vi "FP_Size To Bounds.vi"(8 "Error":errorcluster, 9 "Border Spacing":i16, 10 "Bounds":T2, 11 "VI":refnum<vi>) -> (0 "Error Out":errorcluster, 2 "Front Panel box":T1, 3 "VI Out":refnum<vi>)   [LabVIEW 2024]
uses:
  <vilib>/Utility/miscctls.llb/LVBoundsTypeDef.ctl
  <vilib>/Utility/miscctls.llb/LVRectTypeDef.ctl
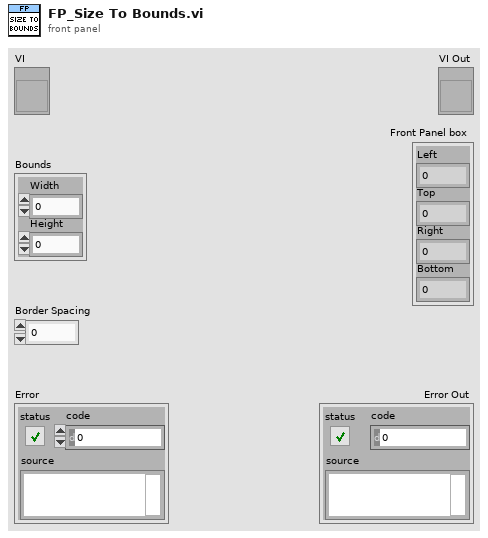
[diagram p1: front panel]
types:
  T1 = typedef "LVRectTypeDef.ctl" = cluster{"Left":i16, "Top":i16, "Right":i16, "Bottom":i16}
  T2 = typedef "LVBoundsTypeDef.ctl" = cluster{"Width":u32, "Height":u32}
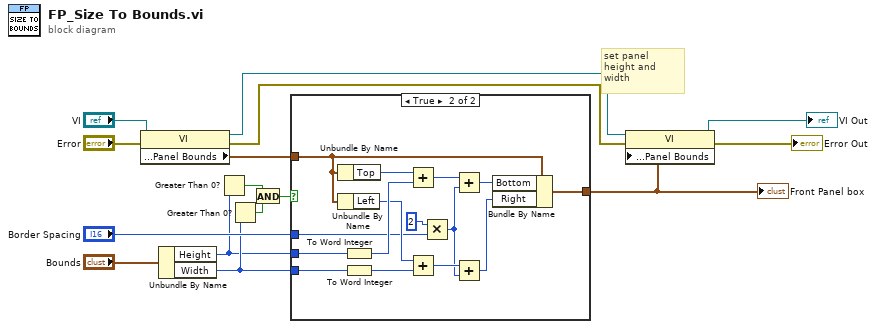
[diagram p0: block diagram]
diagram:
  # "set panel height and width"
  n1 = property on="Property Node" class="VI"(reference="VI", error in="Error") -> (reference out=w7:refnum<vi>, error out=w6:errorcluster, "Front Panel Window:Panel Bounds"=w12:T1)
  n2 = Unbundle By Name("Bounds") -> ("Height"=w4:u32, "Width"=w5:u32)
  n3 = Greater Than 0?(x=w4) -> (x > 0?=w3:bool)
  n4 = Greater Than 0?(x=w5) -> (x > 0?=w2:bool)
  n5 = And(x=w3, y=w2) -> (x .and. y?=w1:bool)
  n6 = case shown="True" w1 {
    tunnel: w4 -> [_ w31]
    tunnel: w5 -> [_ w30]
    tunnel: w12 -> [w16 w21]
    tunnel: "Border Spacing" -> [_ w18]
    tunnel: [w16 w17] -> w9
    frame False {
    }
    frame True {
      n7 = Unbundle By Name(w21) -> ("Top"=w22:i16)
      n8 = Unbundle By Name(w21) -> ("Left"=w23:i16)
      n9 = To Word Integer(number=w31) -> (16bit integer=w26:i16)
      n10 = To Word Integer(number=w30) -> (16bit integer=w27:i16)
      n11 = Add(x=w22, y=w26) -> (x+y=w25:i16)
      n12 = Add(x=w23, y=w27) -> (x+y=w24:i16)
      n13 = Multiply(x=i16 2 ("y"), y=w18) -> (x*y=w19:i16)
      n14 = Add(x=w25, y=w19) -> (x+y=w28:i16)
      n15 = Add(x=w24, y=w19) -> (x+y=w29:i16)
      n16 = Bundle By Name(cluster=w21, "Bottom"=w28, "Right"=w29) -> (w17:T1)
    }
  }
  "Front Panel box" <- w9
  n17 = property on="Property Node" class="VI"(reference=w7, error in=w6, "Front Panel Window:Panel Bounds"=w9) -> (reference out=→"VI Out":refnum<vi>, error out=→"Error Out":errorcluster)
